vi "WS1021 Calc DCAP_RTZ_Percentage.vi"(6 "Cmin(fF)":dbl[](array[numeric]), 8 "Error In":errorcluster, 11 "Input":string[][](table)) -> (0 "Error Out":errorcluster, 1 "% Total Delta C(fF)":string[](array[string]), 2 "Total Delta C(fF)":string[](array[string]), 3 "RTZ (fF)":string[][](array[string]), 5 "% Beam Delta C(fF)":string[][](array[string]), 7 "Delta Cap(fF)":string[][](array[string]))   [LabVIEW 2017]
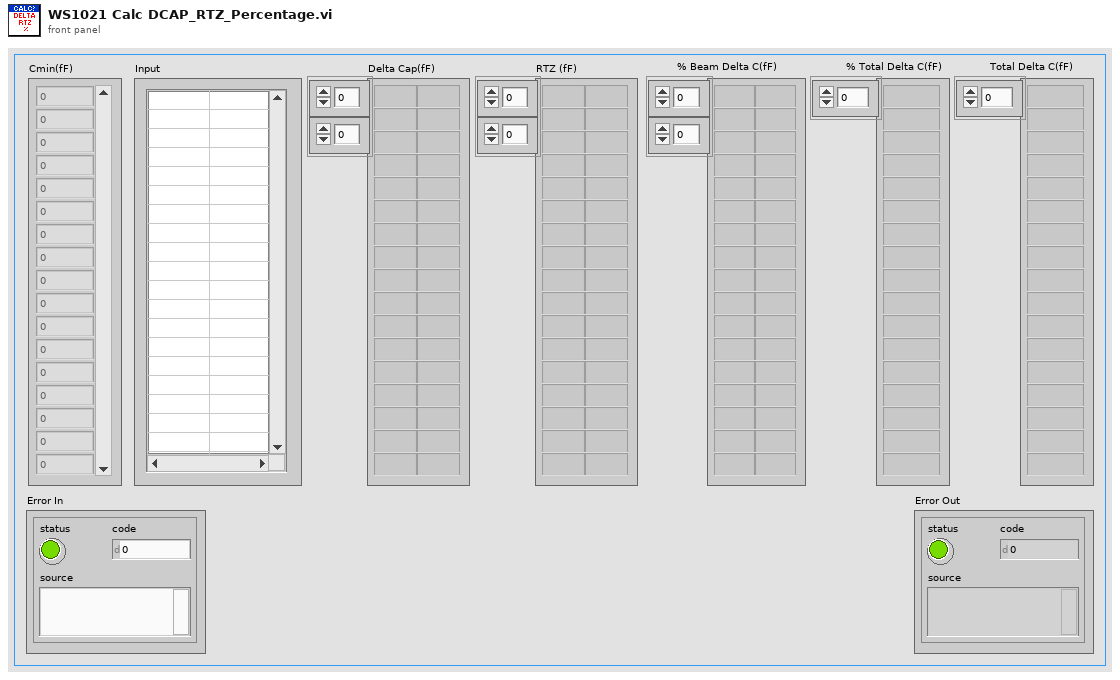
[diagram p1: front panel]
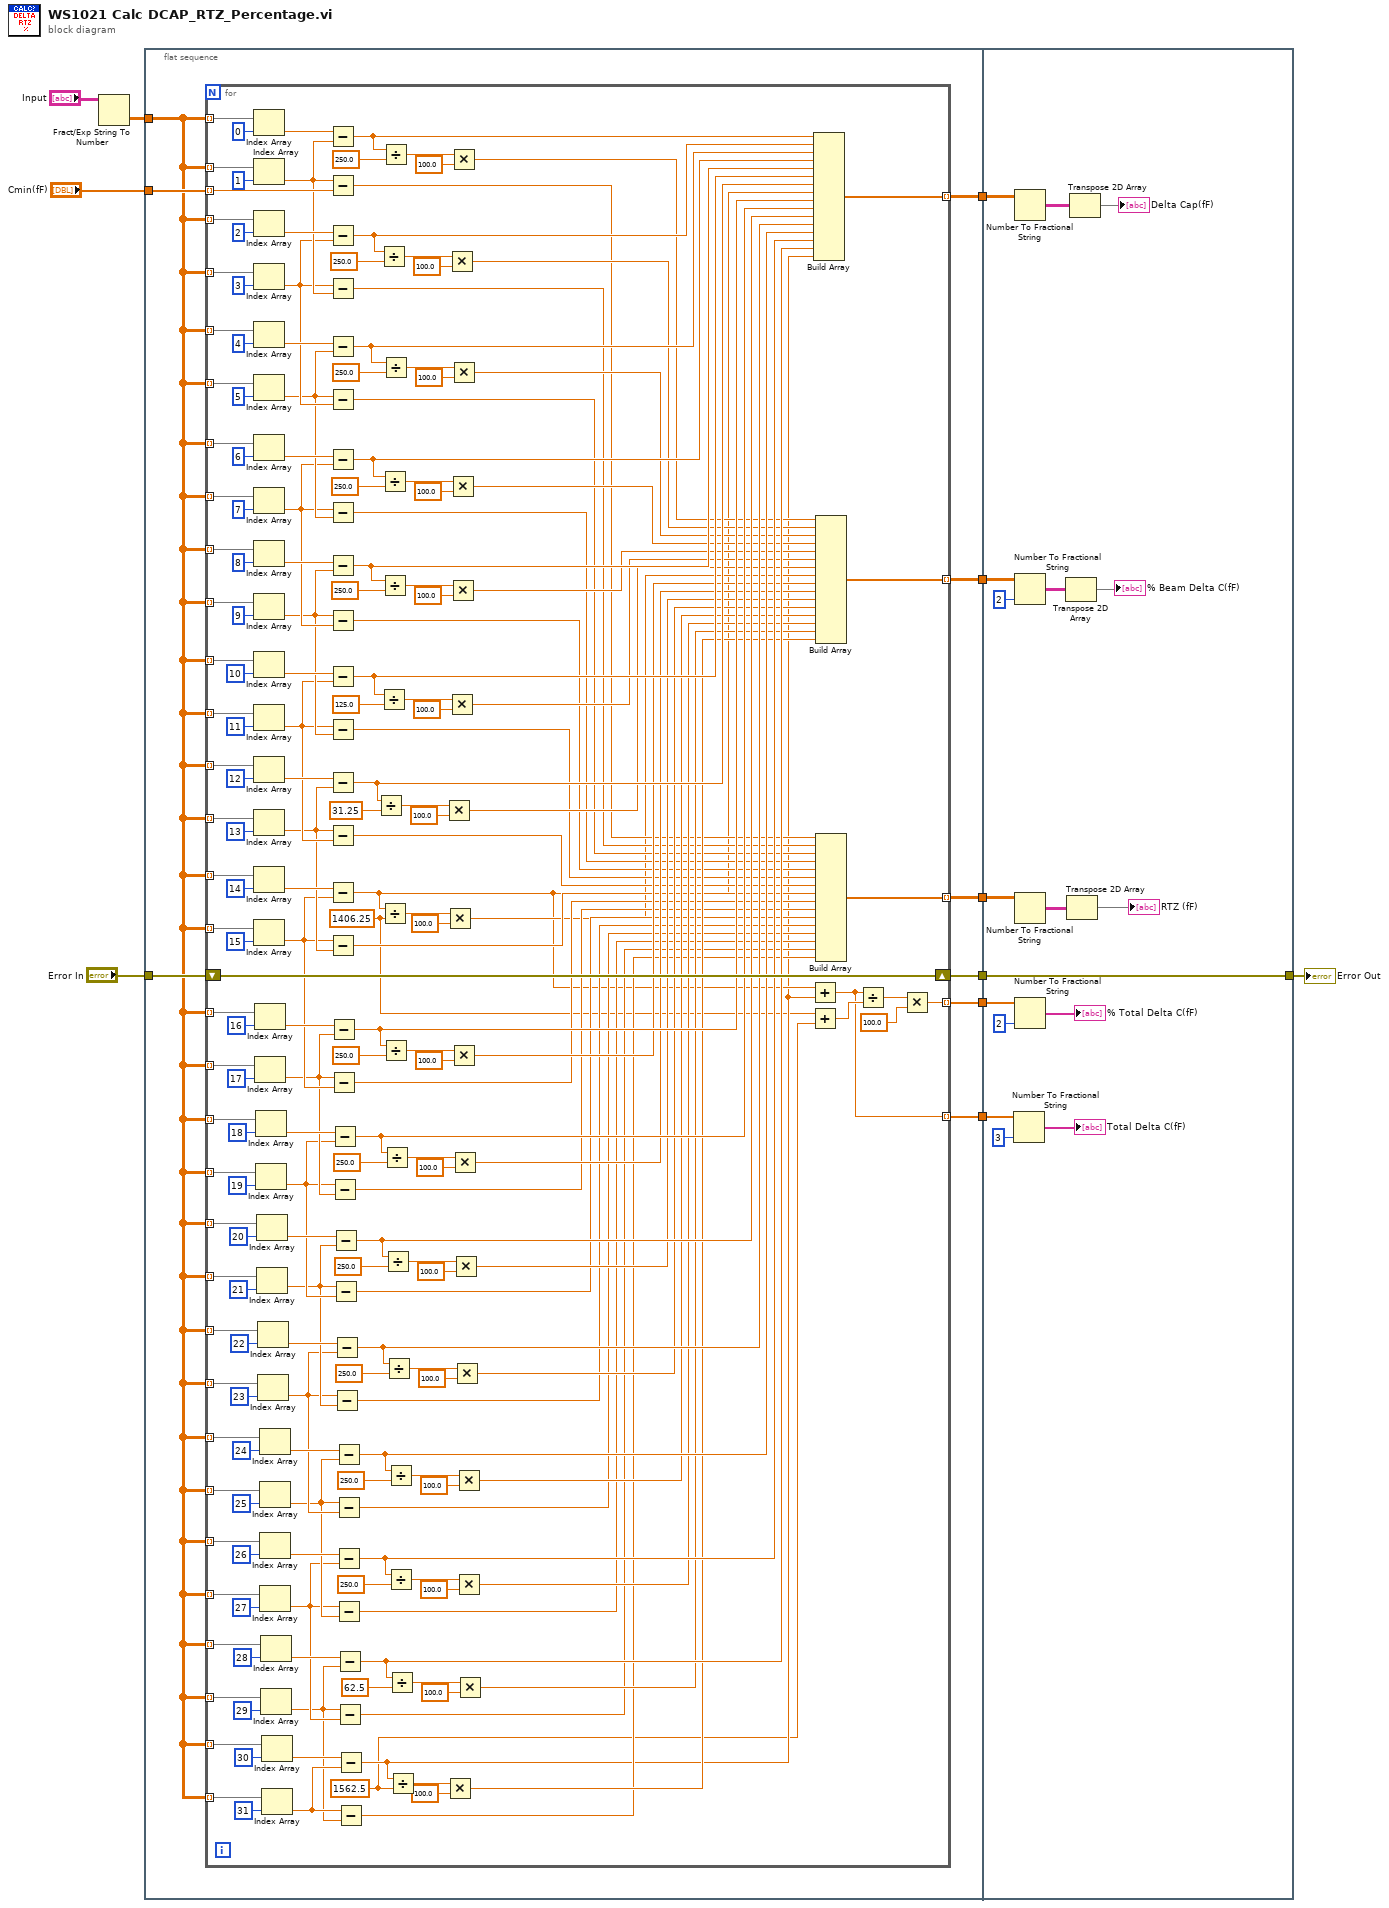
[diagram p0: block diagram]
diagram:
  n1 = Fract/Exp String To Number(string="Input") -> (number=w7:dbl[][])  [unwired: 3 in, 1 out]
  n2 = flat-sequence {
    tunnel: "Error In" -> [w20]
    tunnel: "Cmin(fF)" -> [w18]
    tunnel: w7 -> [w17]
    tunnel: [w19] -> w6
    tunnel: [w16] -> w5
    tunnel: [w15] -> w4
    tunnel: [w14] -> w3
    tunnel: [w13] -> w2
    tunnel: [w12] -> w1
    tunnel: [w239] -> w9
    tunnel: w6 -> [w239]
    tunnel: w5 -> [w238]
    tunnel: w4 -> [w237]
    tunnel: w3 -> [w235]
    tunnel: w2 -> [w233]
    tunnel: w1 -> [w231]
    frame #0 {
      n3 = for {
        tunnel: w17 -> [w219] mode=indexing
        tunnel: w18 -> [w217] mode=indexing
        tunnel: w17 -> [w218] mode=indexing
        tunnel: w17 -> [w214] mode=indexing
        tunnel: w17 -> [w212] mode=indexing
        tunnel: w17 -> [w209] mode=indexing
        tunnel: w17 -> [w208] mode=indexing
        tunnel: w17 -> [w203] mode=indexing
        tunnel: w17 -> [w202] mode=indexing
        tunnel: w17 -> [w198] mode=indexing
        tunnel: w17 -> [w197] mode=indexing
        tunnel: w17 -> [w193] mode=indexing
        tunnel: w17 -> [w192] mode=indexing
        tunnel: w17 -> [w189] mode=indexing
        tunnel: w17 -> [w188] mode=indexing
        tunnel: w17 -> [w183] mode=indexing
        tunnel: w17 -> [w182] mode=indexing
        shift-right: [w181] -> w19
        shift-left: w20 -> [w181]
        tunnel: w17 -> [w146] mode=indexing
        tunnel: w17 -> [w145] mode=indexing
        tunnel: w17 -> [w138] mode=indexing
        tunnel: w17 -> [w137] mode=indexing
        tunnel: w17 -> [w124] mode=indexing
        tunnel: w17 -> [w123] mode=indexing
        tunnel: w17 -> [w122] mode=indexing
        tunnel: w17 -> [w121] mode=indexing
        tunnel: w17 -> [w114] mode=indexing
        tunnel: w17 -> [w113] mode=indexing
        tunnel: w17 -> [w106] mode=indexing
        tunnel: w17 -> [w105] mode=indexing
        tunnel: w17 -> [w98] mode=indexing
        tunnel: w17 -> [w97] mode=indexing
        tunnel: w17 -> [w94] mode=indexing
        tunnel: w17 -> [w93] mode=indexing
        tunnel: [w73] -> w16 mode=indexing
        tunnel: [w50] -> w15 mode=indexing
        tunnel: [w25] -> w13 mode=indexing
        tunnel: [w24] -> w14 mode=indexing
        tunnel: [w23] -> w12 mode=indexing
        w29 = 1562.5 ("y")
        w30 = 1406.25 ("y")
        # "Reg3"
        n4 = Index Array(array=w219, index=0) -> (element=w221:dbl)
        n5 = Index Array(array=w218, index=1) -> (element=w159:dbl)
        n6 = Index Array(array=w214, index=2) -> (element=w215:dbl)
        n7 = Index Array(array=w212, index=3) -> (element=w158:dbl)
        n8 = Index Array(array=w209, index=4) -> (element=w211:dbl)
        n9 = Index Array(array=w208, index=5) -> (element=w157:dbl)
        n10 = Index Array(array=w203, index=6) -> (element=w204:dbl)
        n11 = Index Array(array=w202, index=7) -> (element=w156:dbl)
        n12 = Index Array(array=w198, index=8) -> (element=w201:dbl)
        n13 = Index Array(array=w197, index=9) -> (element=w155:dbl)
        n14 = Index Array(array=w193, index=10) -> (element=w194:dbl)
        n15 = Index Array(array=w192, index=11) -> (element=w154:dbl)
        n16 = Index Array(array=w189, index=12) -> (element=w187:dbl)
        n17 = Index Array(array=w188, index=13) -> (element=w153:dbl)
        n18 = Index Array(array=w183, index=14) -> (element=w186:dbl)
        n19 = Index Array(array=w182, index=15) -> (element=w88:dbl)
        n20 = Index Array(array=w146, index=16) -> (element=w147:dbl)
        n21 = Index Array(array=w145, index=17) -> (element=w87:dbl)
        n22 = Index Array(array=w138, index=18) -> (element=w144:dbl)
        n23 = Index Array(array=w137, index=19) -> (element=w86:dbl)
        n24 = Index Array(array=w124, index=20) -> (element=w130:dbl)
        n25 = Index Array(array=w123, index=21) -> (element=w85:dbl)
        n26 = Index Array(array=w122, index=22) -> (element=w131:dbl)
        n27 = Index Array(array=w121, index=23) -> (element=w84:dbl)
        n28 = Index Array(array=w114, index=24) -> (element=w120:dbl)
        n29 = Index Array(array=w113, index=25) -> (element=w83:dbl)
        n30 = Index Array(array=w106, index=26) -> (element=w107:dbl)
        n31 = Index Array(array=w105, index=27) -> (element=w82:dbl)
        n32 = Index Array(array=w98, index=28) -> (element=w104:dbl)
        n33 = Index Array(array=w97, index=29) -> (element=w81:dbl)
        n34 = Index Array(array=w94, index=30) -> (element=w90:dbl)
        n35 = Index Array(array=w93, index=31) -> (element=w89:dbl)
        n36 = Subtract(x=w221, y=w159) -> (x-y=w80:dbl)
        n37 = Subtract(x=w159, y=w217) -> (x-y=w49:dbl)
        n38 = Subtract(x=w215, y=w158) -> (x-y=w79:dbl)
        n39 = Subtract(x=w158, y=w159) -> (x-y=w48:dbl)
        n40 = Subtract(x=w211, y=w157) -> (x-y=w78:dbl)
        n41 = Subtract(x=w157, y=w158) -> (x-y=w47:dbl)
        n42 = Subtract(x=w204, y=w156) -> (x-y=w77:dbl)
        n43 = Subtract(x=w156, y=w157) -> (x-y=w46:dbl)
        n44 = Subtract(x=w201, y=w155) -> (x-y=w76:dbl)
        n45 = Subtract(x=w155, y=w156) -> (x-y=w45:dbl)
        n46 = Subtract(x=w194, y=w154) -> (x-y=w75:dbl)
        n47 = Subtract(x=w154, y=w155) -> (x-y=w44:dbl)
        n48 = Subtract(x=w187, y=w153) -> (x-y=w74:dbl)
        n49 = Subtract(x=w153, y=w154) -> (x-y=w43:dbl)
        n50 = Subtract(x=w186, y=w88) -> (x-y=w32:dbl)
        n51 = Subtract(x=w88, y=w153) -> (x-y=w42:dbl)
        n52 = Subtract(x=w147, y=w87) -> (x-y=w72:dbl)
        n53 = Subtract(x=w87, y=w88) -> (x-y=w41:dbl)
        n54 = Subtract(x=w144, y=w86) -> (x-y=w71:dbl)
        n55 = Subtract(x=w86, y=w87) -> (x-y=w40:dbl)
        n56 = Subtract(x=w130, y=w85) -> (x-y=w70:dbl)
        n57 = Subtract(x=w85, y=w86) -> (x-y=w39:dbl)
        n58 = Subtract(x=w131, y=w84) -> (x-y=w69:dbl)
        n59 = Subtract(x=w84, y=w85) -> (x-y=w38:dbl)
        n60 = Subtract(x=w120, y=w83) -> (x-y=w68:dbl)
        n61 = Subtract(x=w83, y=w84) -> (x-y=w37:dbl)
        n62 = Subtract(x=w107, y=w82) -> (x-y=w67:dbl)
        n63 = Subtract(x=w82, y=w83) -> (x-y=w36:dbl)
        n64 = Subtract(x=w104, y=w81) -> (x-y=w66:dbl)
        n65 = Subtract(x=w81, y=w82) -> (x-y=w35:dbl)
        n66 = Subtract(x=w90, y=w89) -> (x-y=w31:dbl)
        n67 = Subtract(x=w89, y=w81) -> (x-y=w34:dbl)
        n68 = Divide(x=w74, y=31.25) -> (x/y=w163:dbl)
        n69 = Divide(x=w79, y=250.0) -> (x/y=w175:dbl)
        n70 = Divide(x=w75, y=125.0) -> (x/y=w164:dbl)
        n71 = Divide(x=w77, y=250.0) -> (x/y=w169:dbl)
        n72 = Divide(x=w76, y=250.0) -> (x/y=w168:dbl)
        n73 = Divide(x=w32, y=w30) -> (x/y=w160:dbl)
        n74 = Divide(x=w80, y=250.0) -> (x/y=w179:dbl)
        n75 = Divide(x=w78, y=250.0) -> (x/y=w174:dbl)
        n76 = Divide(x=w72, y=250.0) -> (x/y=w152:dbl)
        n77 = Divide(x=w71, y=250.0) -> (x/y=w139:dbl)
        n78 = Divide(x=w70, y=250.0) -> (x/y=w125:dbl)
        n79 = Divide(x=w69, y=250.0) -> (x/y=w136:dbl)
        n80 = Divide(x=w68, y=250.0) -> (x/y=w115:dbl)
        n81 = Divide(x=w67, y=250.0) -> (x/y=w112:dbl)
        n82 = Divide(x=w66, y=62.5) -> (x/y=w99:dbl)
        n83 = Divide(x=w31, y=w29) -> (x/y=w92:dbl)
        n84 = Multiply(x=w163, y=100.0) -> (x*y=w63:dbl)
        n85 = Multiply(x=w160, y=100.0) -> (x*y=w33:dbl)
        n86 = Multiply(x=w92, y=100.0) -> (x*y=w55:dbl)
        n87 = Multiply(x=w175, y=100.0) -> (x*y=w53:dbl)
        n88 = Multiply(x=w164, y=100.0) -> (x*y=w64:dbl)
        n89 = Multiply(x=w169, y=100.0) -> (x*y=w51:dbl)
        n90 = Multiply(x=w168, y=100.0) -> (x*y=w65:dbl)
        n91 = Multiply(x=w179, y=100.0) -> (x*y=w54:dbl)
        n92 = Multiply(x=w174, y=100.0) -> (x*y=w52:dbl)
        n93 = Multiply(x=w152, y=100.0) -> (x*y=w62:dbl)
        n94 = Multiply(x=w139, y=100.0) -> (x*y=w61:dbl)
        n95 = Multiply(x=w125, y=100.0) -> (x*y=w60:dbl)
        n96 = Multiply(x=w136, y=100.0) -> (x*y=w59:dbl)
        n97 = Multiply(x=w115, y=100.0) -> (x*y=w58:dbl)
        n98 = Multiply(x=w112, y=100.0) -> (x*y=w57:dbl)
        n99 = Multiply(x=w99, y=100.0) -> (x*y=w56:dbl)
        n100 = Add(x=w32, y=w31) -> (x+y=w23:dbl)
        n101 = Add(x=w30, y=w29) -> (x+y=w28:dbl)
        n102 = Build Array(w80, w79, w78, w77, w76, w75, w74, w32, w72, w71, w70, w69, w68, w67, w66, w31) -> (w73:dbl[])
        n103 = Build Array(w54, w53, w52, w51, w65, w64, w63, w33, w62, w61, w60, w59, w58, w57, w56, w55) -> (w50:dbl[])
        n104 = Build Array(w49, w48, w47, w46, w45, w44, w43, w42, w41, w40, w39, w38, w37, w36, w35, w34) -> (w24:dbl[])
        n105 = Divide(x=w23, y=w28) -> (x/y=w27:dbl)
        n106 = Multiply(x=w27, y=100.0) -> (x*y=w25:dbl)
      }
    }
    frame #1 {
      n107 = Number To Fractional String(number=w231, precision (6)=i16 3) -> (F-format string=→"Total Delta C(fF)":string[])  [unwired: 2 in]
      n108 = Number To Fractional String(number=w238) -> (F-format string=w228:string[][])  [unwired: 3 in]
      n109 = Number To Fractional String(number=w237, precision (6)=i16 2) -> (F-format string=w226:string[][])  [unwired: 2 in]
      n110 = Number To Fractional String(number=w235) -> (F-format string=w224:string[][])  [unwired: 3 in]
      n111 = Number To Fractional String(number=w233, precision (6)=i16 2) -> (F-format string=→"% Total Delta C(fF)":string[])  [unwired: 2 in]
      n112 = Transpose 2D Array(2D array=w226) -> (transposed array=→"% Beam Delta C(fF)":string[][])
      n113 = Transpose 2D Array(2D array=w224) -> (transposed array=→"RTZ (fF)":string[][])
      n114 = Transpose 2D Array(2D array=w228) -> (transposed array=→"Delta Cap(fF)":string[][])
    }
  }
  "Error Out" <- w9
